vi "Day 10-2.vi"() -> ()   [LabVIEW 2020]
uses:
  Open Symbol.ctl
  <vilib>/regexp/Match Regular Expression.xnode
panel:
  out "Answer":u64
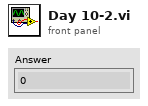
[diagram p1: front panel]
types:
  T1 = typedef "Open Symbol.ctl" = enum16{"(", "[", "{", "<"}
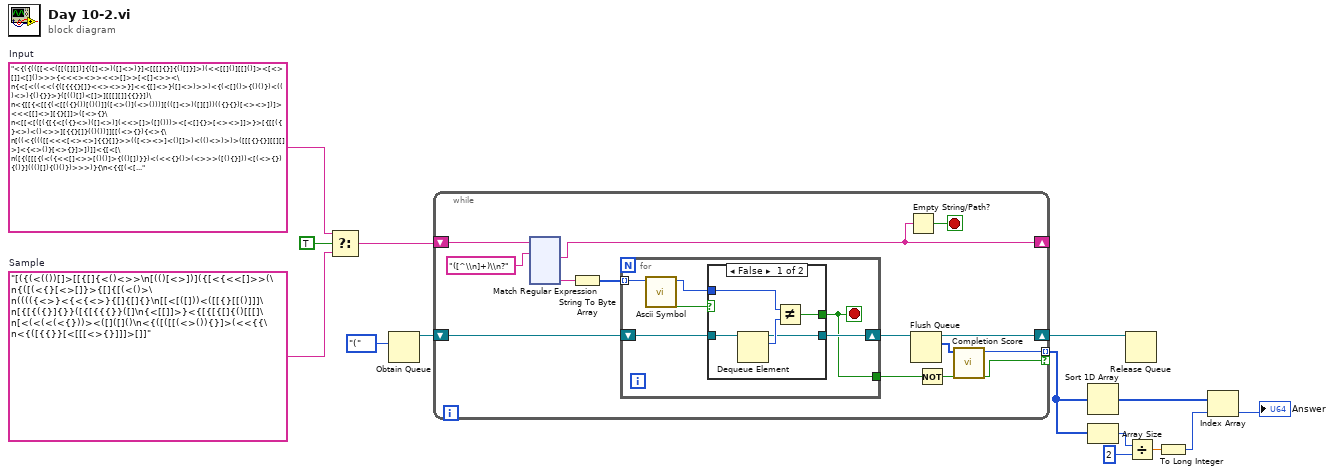
[diagram p0: block diagram]
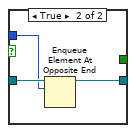
[diagram p2: hidden frame]
diagram:
  w13 = "[({(<(())[]>[[{[]{<()<>>\n[(()[<>])]({[<{<<[]>>(\n{([(<{}[<>[]}>{[]{[(<()>\n(((({<>}<{<{<>}{[]{[]{}\n[[<[([]))<([[{}[[()]]]\n[{[{({}]{}}([{[{{{}}([]\n{<[[]]>}<{[{[{[]{()[[[]\n[<(<(<(<{}))><([]([]()\n<{([([[(<>()){}]>(<<{{\n<{([{{}}[<[[[<>{}]]]>[]]"  # Sample
  w14 = "<{({(([[<<([[([][])]{([]<>)([]<>)}]<[[[]{}]{()[]}]>)(<<[[]()][[]()]><[<>[]]<[]()>>>{<<<><>><<>[]>>[<[]<>><\n{<[<((<<({([{{{}[]}<<><>>}]<<{[]<>}([]<>)>>)<{(<[]()>{()()})<(()<>){(){}}>}([(()[])<[]>][[[][]]{{}}])\n<{[[{<[[{(<[[({}())[()()]]([<>()](<>()))][(([]<>)([][]))(({}{})[<><>])]><<<[[]<>][{}[]]>([<>{}\n<[[<[([({[{<[({}<>)([]<>)](<<>[]>([]()))><[<[]{}>[<><>]]>}>[{[[({}<>)<()<>>][{{}[]}(()())]][[(<>{}){<>{\n[((<{((([[<<<[<><>]{{}[]}>>(([<><>]<()[]>)<(()<>)>)>([[[{}{}][[][]>]<{<>()}[<>{}]>])]]<{[<[\n([{([[[{(<({<<[]<>>[()()]>{(()[])}})<(<<{}()>(<>>>([(){}]))<[(<>{}){()}]((()[]){()()})>>>)}{\n<{{[(<[<<[[{<(()[])>[[{}()]{{}[]}]}[[(<>())[()()]]{<{}{}>}]](<{[<><>]{{}{}}}<({}[])[<><>]>><{[{}<>](<><>)\n{({<[<([[(({({<>()}{{}{}})})<<<((){})[[]()]><{{}()}[[][]]>>{(<{}{}>{{}()})}>)<<{<[{}[]][{}{}]>([[][]]{\n{[(((((<{[({<{()[]}(()())>{<(){}>{{}()}}}(<[<>()]{[]()}>(<()()>{{}<>})))[<[[{}{}](<>()>]({[]<>\n(([((<{<[((<{{<><>}{[]{}}}><<<<>>[{}]>([[]{}]<<>[]>)>)[[{<{}>{()()}}[[{}[]](()()>]](<<<>{}>[[]\n{<([[{<{([[<([[]<>]({}{})){{{}()}({}[])}>](<(<()()><()[]>)<<[]<>>([]{})>>)]){[{<<[()[]]<<>{}>><({\n<{[[([<<<(<{{(()<>)(()())}([{}<>]((){}))}>)>({({{{()<>}({}<>)}<[[]<>]{<>[]}>})(({<(){}>[<>[]]}<([]{})<[]{}>>)\n(<{<{[[({(<[((<>[]){{}})<(<><>)<[]{}>>]((<<>[]><[]()>)<<{}{}>{(){}}>)>(<[[[]<>]]{{<>{}}{[]()}}>(<{\n{(({{[[{<[((<<()<>>[{}{}]>((()<>){[]()})){{(<>{})[<>[]]}<<<><>>>}){{({<>{}}([]()))[{<><>}{[]\n(([<(([({{<{[{()<>}<{}[]>]}{[[()()][()<>]}[{<>{}}({}{})]}>((<<<>{}>[<>()]>{{[]<>}({}{})}){[<{\n[[{{(<<[[[[<<<<>{}>({}())>[([]<>)(()())]>]<<<{<>()}>[<<>[]>[()()]]>[([[]()]<[][]))<[<>{}]{{}<>\n{[{(((([<[{([(()()){()()}][<(){}>[{}<>)])[(<{}<>>{<>()})({{}<>}[()[]])]}(<({[]<>}<()[]>)({[]<>\n<<([(([{<{<<<[{}[]]((){})>((<>[])(()<>))>{{{<>()}{[]}}{([][])}}>[<{{<>[]}<<>>}({[]<>})>]]({({{<><>\n[{((<{<[[<[{[{{}<>}]{[{}][<>[]]}}[<([]())<()[]>>((<>){[]{}})]]<{(<()<>><{}<>]){[[]<>]({}{})}}({<{}[]>{{}\n<[<{(<[[<(((<({}[])><(<><>)(<>())]){{{()()}(<>())}<[{}()]>})[([[<>[]]{{}[]}]{{{}()}<{}[]>})[[(()<>){<>\n[([{{[<([{[([[()<>]])([[<>][()[]]][[<>[]]<<>[]>])]}{([<<{}()>({})>(<[]()>(<><>))]<<{{}<>}{<>}><(<>\n<<[[([([(<(<<[{}[]]<()[]]><{[]{}}[<>()]>>)>[<<({[][]}<<><>>)[<{}{}>{()<>}]><({<>{}}([]))((\n<({<{(<[({([[{()}(<><>)](<[][]>[{}{}])](([[]<>]<<>{}>))){({<<>{}>[[]{}]}<([][])>)<<(<><>)<[]<>>}>}}((([[()<\n{([<(<[(({[({[(){}]<<>{}>}[[{}{}][{}[]]])]{({[()<>]{()[]}}(<[][]>[()[]])){{{[]{}}(<>[])}[<(){}>(\n<[<[<{[{<[{[<<{}<>>(<>)>]{<({}{}){(){}}>((<>{})[{}<>])}}[<[[<><>]{{}<>}]{<()()>}>{<<[]()>(()())>{{{}<\n(({[[<<[({[{{<()()>}}{<[<>()]>}][(<{[][]}>{[{}()]{[]<>}})<{{<>{}}(()[])}{{[]()}<<>[]>}>]})\n<((<([[({(<{[[(){}]<[][]>]}>({<[()<>](()[])>(([]<>)([]<>))}<{[[]<>]{(){}}}(<()<>>([][]])>))}<{[<[({}\n{({{{[[{{[{(<<(){}>[{}{}]>((()<>)[<>{}]))[<<{}[]><[]>>[{{}{}}(<>[])]]}[(<<(){}>({}{}))((<>{})([]<>)))\n[[(({[{(<({[{<[]()>{()[]}}<(<>())<()()>>]<(({}[]){{}<>])((()<>){{}[]})>}([[({}{})[<>()]][{<><>}]]{([[\n[[{<[([<[((<([[]{}][{}<>])([{}<>])>[([()<>]{{}{}}){{[]()}}])<({{[]()}[[]()]))>)([<<<<>{}><{}()>><(<>\n<<({{{<{[<{<{<[]<>>[[]{}]}[<[]()>{[]{}}]>[[[(){}][<><>]]{(<>[]}({}{})}]}><[[({{}[]}{[]()}){(<>())[()<\n{{(({[[[{<[<(([]())([]{}))([{}{}](()[])}>]>}([<{[[[]()][(){}]]<{<>[]}>}({<()<>><[]<>>})>((([()\n(<(({{(([(({{<{}[]>({}())}([<>[]][{}()])}((<[][]>{()<>}){[[]<>]<{}{}>}))<({{[]<>}([][])}{<[]{}>{<>[]}})\n((([<([([{{{<<<>{}><{}[]>>[[<>[]][{}[]]]}}(([<<>{}>[()[]]][{{}{}}])(<[()()][<><>]>{{<>[]}})}}]<{[[<\n{{(<[<[<[<<[[(<>[])]({<><>}[()()])]>>]>[{{[[{(<>[])([][])}{[[][]]([]())}]>[[[<{}{}>({}())]<{<>\n<[{[[([[{[(<[<{}{}>{(){}}][{[]<>}<()[]]]>(([()<>][[][]]){[<>{}](()[])}))[[<<{}>[<>{}]>[({}{})({}{})]]<([[]{}\n({<<<{<({{{{{[()()]({}())}[[[]{}][<><>])}({<()()><[]()>}({<>()}))}{(((<>()){()()}){<(){}><()[]>})(([{}()]\n([<({[{({(<<{[{}()]}{{{}[]}((){})}>>)<<{[((){})[()]]}<<{[]<>}<<>()>>([<>()][[]<>])>>{<<[<>[]]<[]<>>)<{<\n(<[<<(<[[[[{{({}<>)[{}{}]}<[[]{}]([]<>)>}][<[<<>{}>{[]}][[[]{}](<>())]><<[<>()][(){}]><{[]\n(({[[(([<(([{({}[])[<>{}]}{(<>[])({}{})})<<<{}[]>({}())>[({}<>)<{}()>]>)[<<[[][]]((){})><{{}(\n{[((<([<[{[{<[<><>][()()]><{<>{}}>}[{<[][]>[()<>]}<(<>())<()<>>>]]<<<(<>())<()[]>>>[{{{}[]}}[[{}()]((){\n{{<{({{({[<((({}{}){<>[]}){<{}()>{<>[]}})>(<{<<>{}><[]<>>}>[[{[]<>>{<><>}]{((){})<(){}>}])]}(<{[{{<><>}{[\n(({<[[{[(<(((({}{}){()<>}))<{{[]{}}{{}{}}}<[{}<>][(){}]>>)>[{{(<<><>>([]{}))[((){})<{}[]>]}}(([[<>()]{<>()}]\n[<([[[<[<{<{<{[]{}}{[]{}}>[([]())<<>[]>]}({{[]{}}<[]()>}<({}())(<>{})>)>}[({[[{}[]][{}<>]]})]>]><[\n<{[<<[[<{[[{<<{}[]>[<><>]>}({[[]{}]<{}()>}((()[])))]{[<{()}[[]{}]>]{(({}[])<{}()>)<(<>())[()<>]\n[[([[{[[(([{[[<>()]{<>()}]({(){}}({}{}))}[<[<><>]([]())>(<[]()><{}[]>)]]{(<<<><>>[[]{}]>(<[][]>((){}))\n{(<<[[{[{{(<<<{}[]>(<>[])>({[]{}}([]{}))>[{<<>()>[[]<>]]([{}[]])])}[[{(<<><>>[()()])<<<><>>>}([<<>\n([((<(<[(<{((<{}{}>{<><>})){{(()[])[{}[]]}}}{[[[(){}][<><>]]]({<()<>>{{}[]}}<[()()]{()[]}>)}>[<{(<{}\n[(<[([[({({<[{<>()}([]<>)][(<><>)<()[]>]>})[{([(())({}[])][{[]<>}<()<>>])}({<[{}{}](()())><({}())[<>[]\n([(<<[<{<{((<(<>[])({}<>)>{{()()}<<>{}>}))<{[[()[]][()[]]][({}[])<{}()>]}{<({})><{[][]}{{}<>}>}>}<<<({(){}}\n[(<{(([({<{{(<[]<>>({}()))}}[<[[{}[]][[]]]>[({[]<>}(<>{}))]]>})]<([(<([[()()][[][]]]<((){}\n((({([(<<{{<<({}())(())>([<>()]<()()>)>}}<[(<{{}[]}<()<>>><({}{}){(){}}>)][(({()<>}([]()))([()]))({{{}()}\n{<(({[<([{[({([][])[[]{}]}<({}<>)<<>()>>)<<{<>()}{[]<>}>{{{}}{[]()}}>]}])<<{<(([[]{}]<<>[]>)){<<[]<>>><<()[\n[{<(<<<((<<<{[()<>]{[]<>}}>[[<{}{}>[()[]]]<(<><>)[()[]]>]>{[[[[]()][<>[]]]]({(<>}{[]{}}})}>){({\n<<[((<<[{{[(<[<>()]><{{}[]}{<>{}}>){[(()[])([]())][[(){}][{}[]]]}]([<[[][]]{(){}}><<{}{}>{<>{}}>][[\n{<<{<<{<({[[([<>{}])[{[]<>}{{}[]}]][[<()<>>[<>{}]]]]<([{[]()}({}{})]({[]()}{<>()})){[({}<>)[[]{}\n{<<[{((([<([[<[]()><<><>>][{()<>}<[][]>]]{<[{}[]][()[]]>[{<>{}>{[]}]}){[([[]{}]<()[]>)[[<>()][{}[]]\n({{{{<([[((({{{}{}}<()[]>}{<()<>>{{}<>}})(<({}{})>({<>{}}[[]()]))){(<<<><>><()[]>>[{()()}{[]<>}\n({<{[[{({{[<[{[][]}<[][]>]{(<><>)}>([[<>{}][<>{}]]({[]{}}<<>[]>))]}{[({[[]]{()[]}}{(<>{})[()()]})(<{(\n[{<<<[(<(<{((([]{}))[{<>()}[()[]]]){{<{}{}>}[<[]<>>{<>{}}]}}<(<[<>[]][()()]>)<([{}()]{{}[]})\n{{(([[([((<([[<><>]])>({[{()<>}<[]{}>]}<{[()()]<{}>}(<{}<>>({}{}))>))[{{([()()]<{}<>>){(<>{})(\n([(<{[[{<{{<{([]())(<>[])}{{[]<>}{()<>}}>{{{()}}[<[]{}><{}<>>]}}<{[{()()}]{{<>[]}[<><>]}}<<{<>(\n([[{[{[{<<(<{<{}{}>{[]}}{[{}{}]{()[]}}>[{({}[])}<[()[]]>])>>[(<<({<>{}}{[]{}})>>(<[([]()){()<>}]((()())([]\n(({<({<([(({<<<>()>([]())>{<()[]>{[]<>}}}(<{{}<>}[()()]>({{}<>}[{}()]))))]){{<[{[(<>[]){()\n([[(<{[[{<[<(<[]()>[{}[]]){[<><>]{<>[]}}>{{([]()){[]{}}}<((){})([]<>)>}]<<<{{}[]}[()]>(<{}><[][]>)>>>}\n{{(<[{[([<<<[<{}<>>(<>{})]<({}[])[<>[]]>>({<{}{}><[]{}>}<<[]><(){}>>)>>(((({()()}[[]{}]))<[{[]<>)<[]()>]\n(({{<<[{([[({[[]{}]{()<>}}[(<><>)[()()]])[<[<>[]]><([]{})[[][]]>]](<((<><>)<<>()>)[([][])((){})]>[(\n((<<([[<{[{({<(){}><[][]>}{(()[])({}[])})({[{}()]({}{})}(<(){}>(<><>)))}{{[{()<>}<{}{}>][{[]{}}(()\n<{(((([<[((({{{}<>}[[]<>]}<[{}<>]>)[<({}{})>{{[]()}<{}()>}])<([<<>>(<><>)]((()())(<>{})))>){(({(\n<{{<<{{{[({{[<()[]>(()[])]}<<[[]<>][[]]>>}[<[({})<<>[]>][[[]]([][])]>])]}}(<({[[<[(){}]>{<[]{}>}]{(({\n[([[(({([{{({{()}[{}<>]}{({}<>){{}()}}]}}{[<<({}())<(){}>>[{()[]}([]{})]>]{<<{{}()}(<>[])>{[(\n[{[{[([<<((<<{()<>}<<>()>>[{[]{}}{{}[]}]>[[{[][]}{{}}]])(([((){})(()())]{[(){}]{()}})))}{(<<<<<><>>({}[]\n<[{({[({[({{(<[]()>{{}<>}){{{}<>}[(){}]}}(([{}()]<[][]>)[[<>]({}{})])}<<[(<>)({})]<<()[]><\n[((([<(({<<({{{}()}({}<>)}({()[]}[{}{}]))>{[{(<>[])}{(<>[])<{}[]>}]{<[<><>][()[]]>}}>({<{<<>()><<><>>}([{}[]]\n{({((<<([((<[[()[]]{[][]}]<{(){}}{<>{}}>>({[(){}][<>]})))(<(({<>[]}<(){}>)(<()[]><{}()>))>)]){\n<{<[<(<{<[({{{{}<>}<<>{}>}{[[]()][{}{}]}}[({<><>}{<>{}})[[{}()]{[]()}]])({{<[])(<>[])}})](<<[[<><>]](<{}{}>\n[([[[{[((<<(<<()()>>)><<{([]()){<>{}}}<{[]{}}<()()>>>[(<<><>>[()[]]){((){})([]{})}]>>({[<[<><>]{<><\n<{{({{{[<{[{{{()<>}[<><>]}[(()[]){[]{}}]}(<{{}[]}[<>[]]><{{}{}}<{}[]>>)]{(({(){}}<<>{}>)[<<><>>[{}\n[[([[{[({[{[({{}[]}{()[]})[<()()>{{}{}}]][(([]<>)<[][]>)[<{}{}><{}()>]]}][<([([][]){()()}][[{}{}]{()<\n{(<<(((<((((<{()<>}<<>[]>)[<[][]>[{}()]]){[[[]<>]<(){}>][<()<>>{{}<>}]})))<[{{[{{}{}}<[]<>>]}}(\n{[(<{[<{{({[{[<><>](<>{})}{({}[])(<>{})}]}({<({}[])<[]<>>>(({}[]))}[<<()><<>>}[{()[]}{[][]}]])){[({<<>()>(\n<([{[(<(<<([((()())<{}{}>)]<{(<>())(<>()]}{[()<>](<>())}>)<[[<[][]>]{{()}<<><>>}](({()()}[[\n<[<[<{{{[{((<(()()){{}<>)><[[]()](()<>)>))({[[<>{}]{{}()}]({()<>}(()[]))})}]}([{((({{}()}[()<\n[{([({[<(<{[{[<>[]][<>()]}([[]{}](()()))){{[()()]<(){}>}({()[]}<[]()>)}}<{[(<>[]){()<>}][[()<>]{()[]}]}{<(<>\n{((<(<({{([{[([]<>){[]<>}](<[]<>>[[]<>])}{{<[][]><()[]>}({()<>}<<>{}>)}]<[<[<>()]([]{})><{{}<>}<{}<>>>][(\n{<<([<(<{[[{{{<>[]}[[]<>]}{[{}[]]]}{<[(){}]>{[{}()]{[]<>}}}](<{[[]<>]{<>[]}}<<()<>>[[]()]>>)]<[{{<{}>[{}]}<(\n[[{{{<{[{({<<<[]{}>[()<>]><[[]<>]([]<>)>><{<<>()>[<>{}]}>}((<[{}{}]{[]}]{<[]<>>{<>{}}})[([<>(\n[[{<<{{[(([[[{()[]}][[()[]]<[]>]]({{{}}})][({([][])[{}{}]}<[(){}]<()[]>>){<{[]{}}[(){}]><{{}{}}<<>()>]}]))<<\n[(({[<<{<({<([<><>])[{<>()>{{}[]}]>((<()<>><{}<>>)[{[][]}([]{})])})<{{([[]<>]<{}<>>)([()[]]{()()}\n[([(({(<[<[<((<>{})[[]<>]){[<><>]({}[]>}>]>]>)}[(({(<<[{(){}}[()[]]]>[<(<>{}){{}{}}>[[()<>][()]]]>)\n{<{{<({<{((<{({})<<>{}>}((()){()<>})>))}((<{((()[]){{}[]})[<<>>[[]<>]]}(([<>](()<>)))><{{{<>()}((){}}}((\n<[<{<((({{[<{{[][]}}<([]<>)(<>{})>>]}[(([{()()}{<>()}])[<[()[]][()[]]>]){<<[<>()](<>{})>{{(){}}(<>\n(([{([{[<(<(((()<>))[(())(<>{})])([[{}<>]{{}[]}][{<><>}[{}{}]])>[(([()[]]<[][]>)[{{}[]}(()[])])(([{}{}]\n{<(<<{<[{<{<<<<>[]>[[]<>]){[[]()][<><>]}>({(<><>)(()<>)})}>[<([{{}{}}<[]<>>])({{[]<>}({}[])})>]}{<<[(\n<{([({{{<{[{(([]())<<><>>)<[()()]((){})>}]}(<{(<(){}>(<>()))}([[()[]][(){}]](<<>{}>[{}()])}>)>([{<(\n((([{<<[{{[(<<[]<>>(<>())>{({}{})<{}[]>})[[<()()>[<>[]]][<{}[]>(()())]]]}}]>>)]{{{{[[{[[[([]<>){\n({(<{{({[[{<<(()[])[()]>[{<><>}{<>[]}]>{<{<><>}{()[]}>{[{}()]{[][]}}}}{<<{[]<>}(<><>)>{{[]{}}[\n(<[{{(([<{{(<[<>()]((){})>{<{}[]>({}())})}}>][<[{{([{}[]])<([]<>)<<>{}>>}}{<({[][]}(()()))(<<>()>{\n(<<{{{((<{({<<{}()><{}{}>><<()[]>[<>[]]>>(<[(){}]([]<>)>[({}<>)]))(({{[]<>}<()<>>}[<()[]>(()[])]){<[\n<[(((<({([({{[[]()]{[]()}}([{}()]<[]<>>)}[[<()[]>{{}{}}]([<>]<<>()>)]){[((()<>){<>[]}){[{}[]){[\n(({[[({{{[{{({(){}}{{}[]})<({}[])([]<>)>}[[(<>{})]<([]()){{}()}>]}[{<{[]<>}<()()>>([{}<>]<{\n<[({{[<[{({[({[]<>}{{}[]})[{[][]}{[][]}]][[<{}[]>{[]()}]([()[]]({}<>))]}{<{[{}<>]<[]()>}<<[]()>[<>{}]>><((\n[{[{<{{[<<[[<<{}<>>>][{{{}[]}({}())}]]([{<<><>>({}{})}{{[]<>}}]{{{[]()}([]<>)}})><({{<[][]>}}){<{{()><()>}>[<\n{{({([<({(<[({{}{}}<[]{}>)]>[(((<>()){<>()]))[<({}[])(<>{})>{<<><>>{[]()}}]]){{[<(()[])<()<>>>(<()<>>)]([<{}\n[({[<(<<[{<({<{}()>{{}()}})({({})<()()>}[{[]<>}[{}{}]})><[(({}{}))(((){})[[][]])]>}<{([<[]<>>]<[{}[]]((\n[<{{{<<(<[[{<([][]){<>}>}{<[[]]{[]{}}><{<>{}}>}]<<{([]())[<>[]]}><(([]{}){[]<>})[(<>())({}<>}]>>]("  # Input
  n1 = Select(t=w14, s=TRUE, f=w13) -> (s? t:f=w11:string)
  n2 = Obtain Queue(element data type=Open_Symbol."(" ("Open Symbol")) -> (queue out=w9:refnum<queue>)  [unwired: 4 in, 2 out]
  n3 = while {
    shift-right: [w25] -> _
    shift-left: w11 -> [w27]
    shift-right: [w19] -> w8
    shift-left: w9 -> [w21]
    tunnel: [w17] -> w7 mode=indexing if=w15
    stop <- w24 stop-if-true
    n4 = xnode "Match Regular Expression"("input string"=w27, "regular expression"="([^\\n]+)\\n?") -> ("after match"=w25:string, "submatch 1"=w23:string)  [unwired: 4 in, 4 out]
    n5 = String To Byte Array(string=w23) -> (unsigned byte array=w22:u8[])
    n6 = for {
      tunnel: w22 -> [w33] mode=indexing
      shift-right: [w29] -> w20
      shift-left: w21 -> [w30]
      tunnel: [w28] -> w16
      stop <- w28 stop-if-true
      n7 = call "Ascii Symbol.vi"("Character"=w33) -> ("Symbol"=w31:T1, "Open"=w32:bool)  [unwired: 9 in]
      n8 = case shown="False" w32 {
        tunnel: w31 -> [w36 w40]
        tunnel: w30 -> [w38 w41]
        tunnel: [w34 w39] -> w29
        tunnel: [w35 _] -> w28
        frame False {
          n9 = Dequeue Element(queue=w38) -> (queue out=w34:refnum<queue>, element=w37:T1)  [unwired: 2 in, 2 out]
          n10 = Not Equal?(x=w36, y=w37) -> (x != y?=w35:bool)
        }
        frame True {
          n11 = Enqueue Element At Opposite End(queue=w41, element=w40) -> (queue out=w39:refnum<queue>)  [unwired: 2 in, 2 out]
        }
      }
    }
    n12 = Empty String/Path?(string/path=w25) -> (empty?=w24:bool)
    n13 = Flush Queue(queue=w20) -> (queue out=w19:refnum<queue>, remaining elements=w18:T1[])  [unwired: 1 in, 1 out]
    n14 = Not(x=w16) -> (.not. x?=w15:bool)
    n15 = call "Completion Score.vi"("Symbols"=w18) -> ("Score"=w17:u64)  [unwired: 10 in]
  }
  n16 = Sort 1D Array(array=w7) -> (sorted array=w4:u64[])
  n17 = Array Size(array=w7) -> (size(s)=w6:i32)
  n18 = Release Queue(queue=w8) -> ()  [unwired: 2 in, 3 out]
  n19 = Divide(x=w6, y=2) -> (x/y=w1:dbl)
  n20 = To Long Integer(number=w1) -> (32bit integer=w3:i32)
  n21 = Index Array(array=w4, index=w3) -> (element=→"Answer":u64)
